vi "format datetime 1ms.vi"(3 "time stamp":timestamp) -> (1 "datetime string":string)   [LabVIEW 2019, in "Timers.lvlib"]
uses:
  Timers.lvlib
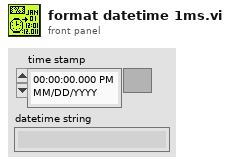
[diagram p1: front panel]
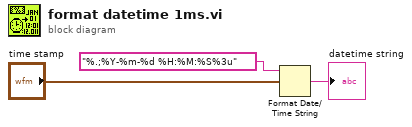
[diagram p0: block diagram]
diagram:
  n1 = Format Date/Time String(time format string (%c)="%.;%Y-%m-%d %H:%M:%S%3u", seconds (now)="time stamp") -> (date/time string=→"datetime string":string)  [unwired: 1 in]
